vi "CRYPEAQ Spectrum.vi"(8 "Freq":dbl format="%0.2f", 10 "Fs":dbl format="%0.2f", 11 "X":dbl[](array[numeric])) -> (0 "Freq":dbl[](array[numeric]), 1 "dF":dbl, 2 "dBSPL Spectrum":dbl[](array[numeric]) format="%.2f", 4 "FFT Size":dbl format="%0.2f")   [LabVIEW 2013]
uses:
  <vilib>/Analysis/4window.llb/windowTd.ctl
  <vilib>/Analysis/2dsp.llb/Real FFT.vi
  <vilib>/Analysis/0measdsp.llb/Scaled Time Domain Window (DBL).vi
  <vilib>/Analysis/2dsp.llb/Zero Padder (DBL).vi
  <vilib>/Analysis/NI_AALPro.lvlib
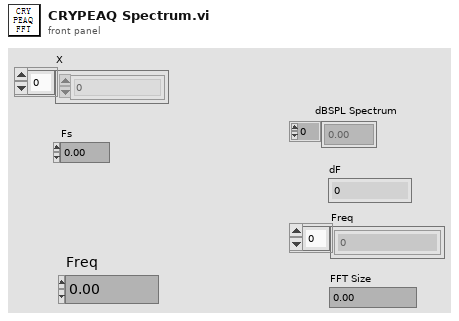
[diagram p1: front panel]
types:
  T1 = typedef "NI_AALPro.lvlib/windowTd.ctl" = u32
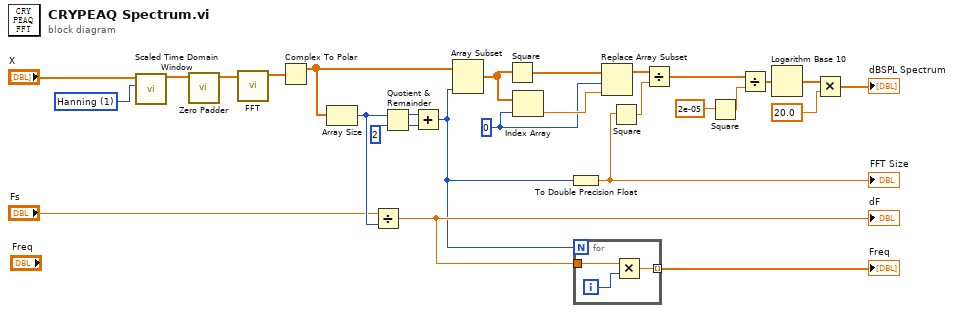
[diagram p0: block diagram]
diagram:
  w26 = 0
  w28 = T1 1 items=["Rectangle"=0, "Hanning"=1, "Hamming"=2, "Blackman-Harris"=3, "Exact Blackman"=4, "Blackman"=5, "Flat Top"=6, "4 Term B-Harris "=7, "7 Term B-Harris"=8, "Low Sidelobe"=9, "Blackman Nuttall"=11, "Triangle"=30, "Bartlett-Hanning"=31, "Bohman"=32, "Parzen"=33, "Welch"=34, "Kaiser"=60, "Dolph-Chebyshev"=61, "Gaussian"=62] ("window")
  n1 = call-poly <vilib>:"Scaled Time Domain Window.vi"("window"=w28, "X"="X") -> ("Windowed X"=w2:dbl[])  [unwired: 7 in, 2 out]
  n2 = call-poly <vilib>:"Zero Padder.vi"("Input Array"=w2) -> ("Zero Padded Array"=w1:dbl[])  [unwired: 10 in]
  n3 = call-poly <vilib>:"FFT.vi"("X"=w1) -> ("FFT {X}"=w15:cdb[])  [unwired: 9 in, 1 out]
  n4 = Complex To Polar(r * e^(i*theta)=w15) -> (r=w19:dbl[])  [unwired: 1 out]
  n5 = Array Size(array=w19) -> (size(s)=w21:i32)
  n6 = Divide(x="Fs", y=w21) -> (x/y=w23:dbl)
  "dF" <- w23
  n7 = Quotient & Remainder(x=w21, y=2) -> (x-y*floor(x/y)=w24:i32, floor(x/y)=w20:i32)
  n8 = Add(x=w24, y=w20) -> (x+y=w7:i32)
  n9 = Array Subset(array=w19, length=w7) -> (w16:dbl[])  [unwired: 1 in]
  n10 = Square(x=w16) -> (x^2=w10:dbl[])
  n11 = Index Array(array=w16, index=w26) -> (element=w27:dbl)
  n12 = To Double Precision Float(number=w7) -> (double precision float=w13:dbl)
  "FFT Size" <- w13
  n13 = for {
    N: w7 -> [_]
    tunnel: w23 -> [w31]
    tunnel: [w30] -> w18 mode=indexing
    i -> [w29]
    n14 = Multiply(x=w31, y=w29) -> (x*y=w30:dbl)
  }
  "Freq" <- w18
  n15 = Replace Array Subset(array=w10, new element=w27, index=w26) -> (w5:dbl[])
  n16 = Square(x=w13) -> (x^2=w12:dbl)
  n17 = Divide(x=w5, y=w12) -> (x/y=w14:dbl[])
  n18 = Square(x=2e-05 ("dB ref.")) -> (x^2=w8:dbl)
  n19 = Divide(x=w14, y=w8) -> (x/y=w6:dbl[])
  n20 = Logarithm Base 10(1:w6) -> (0:w17:dbl[])
  n21 = Multiply(x=w17, y=20.0) -> (x*y=→"dBSPL Spectrum":dbl[])
